vi "UDMA_CHANGE_CB.vi"(0 "TCP Network Connection in":refnum<k5>, 2 "CB_ID":u32=100, 5 "error in (no error)":errorcluster) -> (14 "TCP Network Connection out":refnum<k5>, 17 "STATUS":u32, 19 "error out":errorcluster)   [LabVIEW 2019]
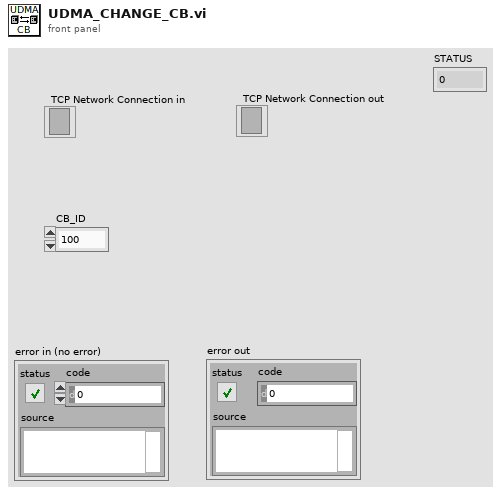
[diagram p1: front panel]
types:
  T1 = enum16{"big-endian, network order", "native, host order", "little-endian"}
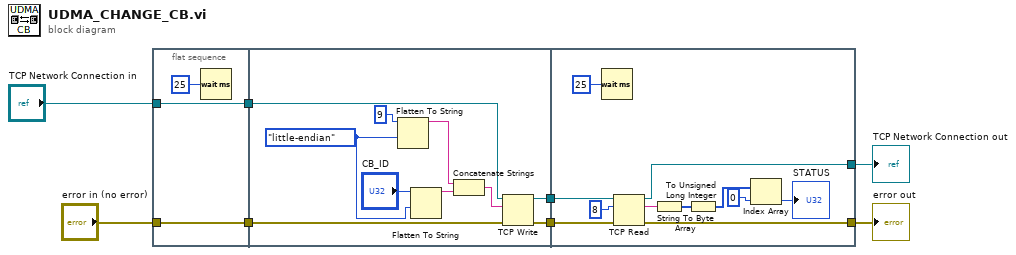
[diagram p0: block diagram]
diagram:
  n1 = flat-sequence {
    tunnel: [w10] -> w4
    tunnel: [w11] -> w3
    tunnel: "error in (no error)" -> [w11]
    tunnel: "TCP Network Connection in" -> [w10]
    tunnel: w4 -> [w21]
    tunnel: w3 -> [w20]
    tunnel: [w19] -> w2
    tunnel: [w18] -> w1
    tunnel: [w29] -> w6
    tunnel: [w30] -> w5
    tunnel: w2 -> [w32]
    tunnel: w1 -> [w31]
    frame #0 {
      n2 = Wait (ms)(milliseconds to wait=u32 25) -> ()  [unwired: 1 out]
    }
    frame #1 {
      w12 = T1."little-endian" ("byte order (0:big-endian, network order)")
      n3 = Flatten To String(anything=u32 9 ("element"), byte order (0:big-endian, network order)=w12) -> (data string=w15:string)  [unwired: 2 in, 2 out]
      n4 = Flatten To String(anything="CB_ID", byte order (0:big-endian, network order)=w12) -> (data string=w17:string)  [unwired: 2 in, 2 out]
      n5 = Concatenate Strings(w15, w17) -> (w14:string)
      n6 = TCP Write(connection ID=w21, data in=w14, error in (no error)=w20) -> (connection ID out=w19:refnum<k5>, error out=w18:errorcluster)  [unwired: 1 in, 1 out]
    }
    frame #2 {
      n7 = Wait (ms)(milliseconds to wait=u32 25) -> ()  [unwired: 1 out]
      n8 = TCP Read(connection ID=w32, bytes to read=8, error in (no error)=w31) -> (connection ID out=w30:refnum<k5>, data out=w26:string, error out=w29:errorcluster)  [unwired: 2 in]
      n9 = String To Byte Array(string=w26) -> (unsigned byte array=w25:u8[])
      n10 = To Unsigned Long Integer(number=w25) -> (unsigned 32bit integer=w24:u32[])
      n11 = Index Array(array=w24, index=0) -> (element=→"STATUS":u32)
    }
  }
  "error out" <- w6
  "TCP Network Connection out" <- w5
